vi "get_ROI_boundary.vi"(8 "error in (no error)":errorcluster, 10 "number of particles":i32, 11 "image in":T2) -> (0 "error out":errorcluster, 2 "points":T1[](array[typedef]))   [LabVIEW 2010]
uses:
  <vilib>/vision/Image Controls.llb/IMAQ Image.ctl
  point_cluster.ctl
  <vilib>/vision/NI_Vision_Development_Module.lvlib
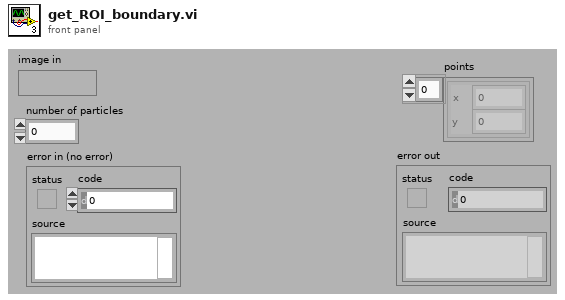
[diagram p1: front panel]
types:
  T1 = typedef "point_cluster.ctl" = cluster{"x":i32, "y":i32}
  T2 = typedef "IMAQ Image.ctl" = refnum<image>
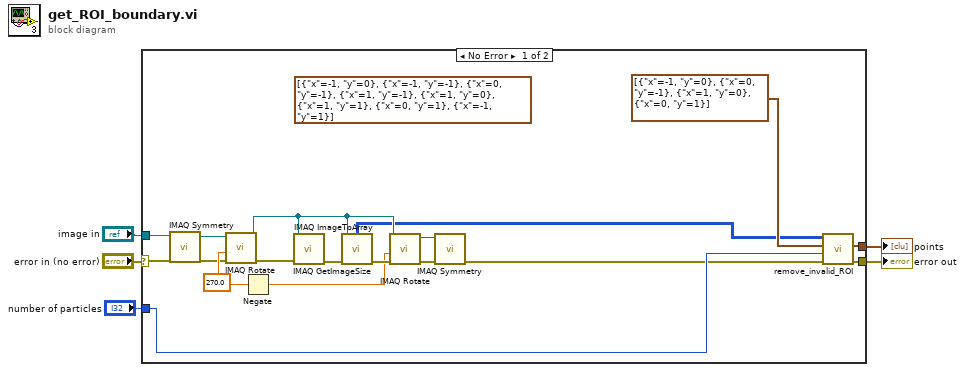
[diagram p0: block diagram]
diagram:
  n1 = case shown="No Error" "error in (no error)" {
    selector: "error in (no error)" -> [w17 w24]
    tunnel: [w11 w24] -> w4
    tunnel: "image in" -> [w15 _]
    tunnel: [w10 _] -> w2
    tunnel: "number of particles" -> [w8 _]
    frame No Error {
      w19 = sgl 270.0 ("Angle (degrees)")
      (unwired) T1[] [{"x"=-1, "y"=0}, {"x"=-1, "y"=-1}, {"x"=0, "y"=-1}, {"x"=1, "y"=-1}, {"x"=1, "y"=0}, {"x"=1, "y"=1}, {"x"=0, "y"=1}, {"x"=-1, "y"=1}]
      n2 = call "IMAQ Symmetry"("error in (no error)"=w17, "Image Src"=w15) -> ("error out"=w16:errorcluster, "Image Dst Out"=w14:T2)  [unwired: 3 in]
      n3 = call "IMAQ Rotate"("error in (no error)"=w16, "Angle (degrees)"=w19, "Image Src"=w14) -> ("error out"=w22:errorcluster, "Image Dst Out"=w20:T2)  [unwired: 7 in]
      n4 = Negate(x=w19) -> (-x=w18:sgl)
      n5 = call "IMAQ GetImageSize"("Image"=w20, "error in (no error)"=w22) -> ("error out"=w23:errorcluster)  [unwired: 2 in, 2 out]
      n6 = call "IMAQ ImageToArray"("error in (no error)"=w23, "Image"=w20) -> ("error out"=w21:errorcluster, "Image Pixels (U8)"=w6:u8[][])  [unwired: 2 in, 3 out]
      n7 = call "IMAQ Rotate"("error in (no error)"=w21, "Angle (degrees)"=w18, "Image Src"=w20) -> ("error out"=w13:errorcluster, "Image Dst Out"=w12:T2)  [unwired: 7 in]
      n8 = call "IMAQ Symmetry"("error in (no error)"=w13, "Image Src"=w12) -> ("error out"=w7:errorcluster)  [unwired: 3 in, 1 out]
      n9 = call "remove_invalid_ROI.vi"("error in (no error)"=w7, "number of particles"=w8, "neighborhood array"=T1[] [{"x"=-1, "y"=0}, {"x"=0, "y"=-1}, {"x"=1, "y"=0}, {"x"=0, "y"=1}], "Image Pixels in"=w6) -> ("error out"=w11:errorcluster, "ROI array out"=w10:T1[])  [unwired: 5 in, 1 out]
    }
    frame Error {
    }
  }
  "points" <- w2
  "error out" <- w4
